vi "Initialize and Register Sessions.vi"(8 "error in":errorcluster, 11 "sequence context":refnum<k7>) -> (0 "error out":errorcluster)   [LabVIEW 2025, in "Session Management xnetCAN.lvlib"]
uses:
  Session Management xnetCAN.lvlib
  <vilib>/gRPC/Generated APIs/ni/measurementlink/sessionmanagement/v1/RPC Messages/ni_measurementlink_PinMapContext.ctl
  <vilib>/Plug-In SDKs/Clients/Session Management V1/Session Reservation/Initialize and Close Session Behavior.ctl
  <vilib>/gRPC/Generated APIs/ni/measurementlink/sessionmanagement/v1/ni.measurementlink.sessionmanagement.v1.api.lvlib
  <vilib>/Plug-In SDKs/Clients/Session Management V1/Session Reservation/Session Reservation.lvclass
  <vilib>/Plug-In SDKs/TestStand/NI Pin Map TestStand.lvlib
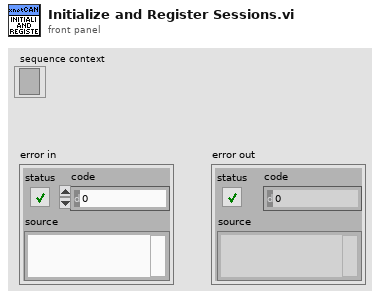
[diagram p1: front panel]
types:
  T1 = typedef "NI Session Management V1 Client.lvlib/Session Reservation.lvclass/Initialize and Close Session Behavior.ctl" = enum16{"Auto", "Initialize and Close", "Attach and Detach", "Initialize and Detach", "Attach and Close"}
  T2 = typedef "ni.measurementlink.sessionmanagement.v1.api.lvlib/ni_measurementlink_PinMapContext.ctl" = cluster{"pin_map_id":string, "sites":i32[]}
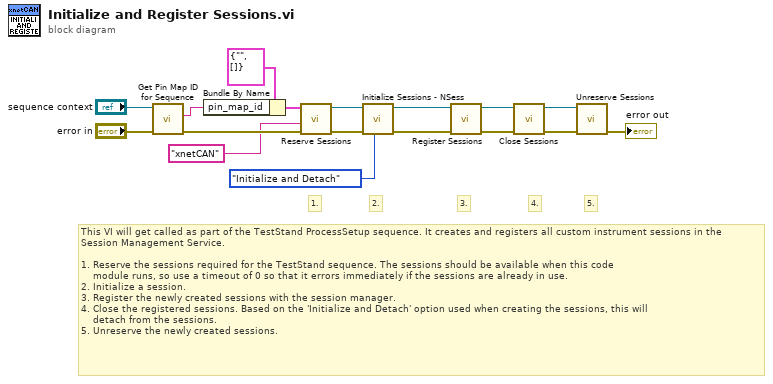
[diagram p0: block diagram]
diagram:
  # "5."
  # "4."
  # "3."
  # "2."
  # "1."
  # "This VI will get called as part of the TestStand ProcessSetup sequence. It creates and registers all custom instrument sessions in the\nSession Management Service.\n\n1. Reserve the sessions required for the TestStand sequence. The sessions should be available when this code\n    module runs, so use a timeout of 0 so that it errors immediately if the sessions are already in use.  \n2. Initialize a session.\n3. Register the newly created sessions with the session manager.\n4. Close the registered sessions. Based on the 'Initialize and Detach' option used when creating the sessions, this will\n    detach from the sessions.\n5. Unreserve the newly created sessions."
  n1 = call <vilib>:"Get Pin Map ID for Sequence.vi"("error in"="error in", "sequence context in"="sequence context") -> ("error out"=w13:errorcluster, "pin map id"=w12:string)  [unwired: 7 in, 1 out]
  n2 = Bundle By Name(cluster=T2 {"pin_map_id"="", "sites"=[]} ("pin map context"), "pin_map_id"=w12) -> (w14:T2)
  n3 = call <vilib>:"Reserve Sessions.vi"("error in"=w13, "instrument type id"="xnetCAN", "pin map context"=w14) -> ("error out"=w4:errorcluster, "session reservation out"=w2:refnum<class "Session Reservation.lvclass">)  [unwired: 7 in]
  n4 = call "Initialize Sessions - NSess.vi"("initialize and close session behavior"=Initialize_and_Close_Session_Behavior."Initialize and Detach", "error in"=w4, "session reservation in"=w2) -> ("error out"=w3:errorcluster, "session reservation out"=w1:refnum<class "Session Reservation.lvclass">)  [unwired: 5 in, 2 out]
  n5 = call <vilib>:"Register Sessions.vi"("error in"=w3, "session reservation in"=w1) -> ("error out"=w8:errorcluster, "session reservation out"=w10:refnum<class "Session Reservation.lvclass">)  [unwired: 8 in]
  n6 = call <vilib>:"Close Sessions.vi"("error in"=w8, "session reservation in"=w10) -> ("error out"=w7:errorcluster, "session reservation out"=w9:refnum<class "Session Reservation.lvclass">)  [unwired: 8 in]
  n7 = call <vilib>:"Unreserve Sessions.vi"("error in"=w7, "session reservation in"=w9) -> ("error out"=→"error out":errorcluster)  [unwired: 9 in]
